vi "ListboxItemsCpr(SubVI).vi"(8 "error in (no error)":errorcluster, 11 "LstBox Refnum":refnum<vi>) -> (0 "error out":errorcluster, 3 "FirstCpr":string)   [LabVIEW 2013, in "main.lvlib"]
uses:
  main.lvlib
  Globals/DataPathGlobalVariable.vi
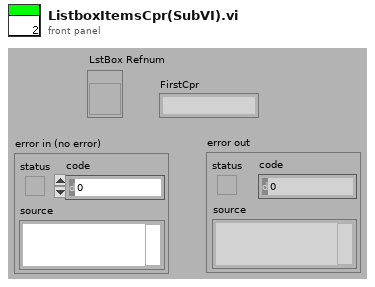
[diagram p1: front panel]
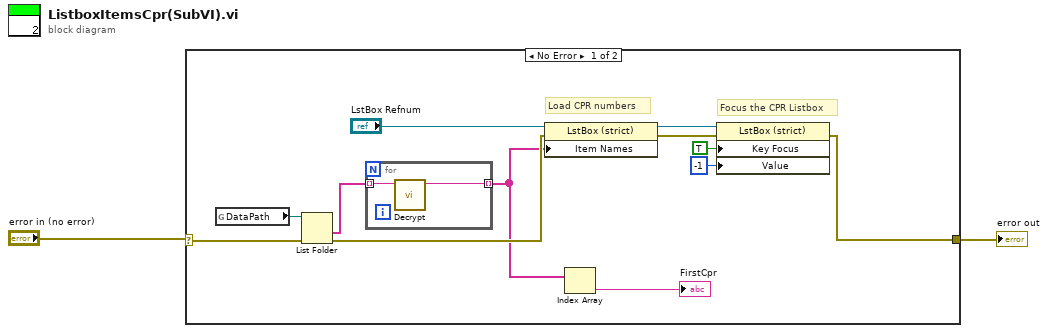
[diagram p0: block diagram]
diagram:
  n1 = case shown="No Error" "error in (no error)" {
    selector: "error in (no error)" -> [w3 w17]
    tunnel: [w8 w17] -> w2
    frame No Error {
      # "Load CPR numbers"
      # "Focus the CPR Listbox"
      n2 = global read "DataPathGlobalVariable.vi" "DataPath"() -> (w12:path)
      n3 = List Folder(path=w12, error in=w3) -> (folder names=w5:string[], error out=w13:errorcluster)  [unwired: 2 in, 2 out]
      n4 = for {
        tunnel: w5 -> [w16] mode=indexing
        tunnel: [w15] -> w4 mode=indexing
        n5 = call "Decrypt.vi"("Input"=w16) -> ("Output"=w15:string)  [unwired: 10 in]
      }
      n6 = property class="LstBox (strict)"(reference="LstBox Refnum", error in=w13, "Item Names"=w4) -> (reference out=w11:refnum<vi>, error out=w9:errorcluster)
      n7 = Index Array(array=w4) -> (element=→"FirstCpr":string)  [unwired: 1 in]
      n8 = property class="LstBox (strict)"(reference=w11, error in=w9, "Key Focus"=TRUE, "Value"=-1 ("Value (Signaling)")) -> (error out=w8:errorcluster)  [unwired: 1 out]
    }
    frame Error {
    }
  }
  "error out" <- w2
